vi "invert joystick cluster values.vi"(6 "Invert Z":bool, 8 "Invert Y":bool, 9 "Invert X":bool, 10 "Slide":cluster{u32, u32, u32}(slide) scale=0.0..7.0, 11 "Joystick Readings":T1) -> (3 "Joystick Readings 2":T1)   [LabVIEW 2012]
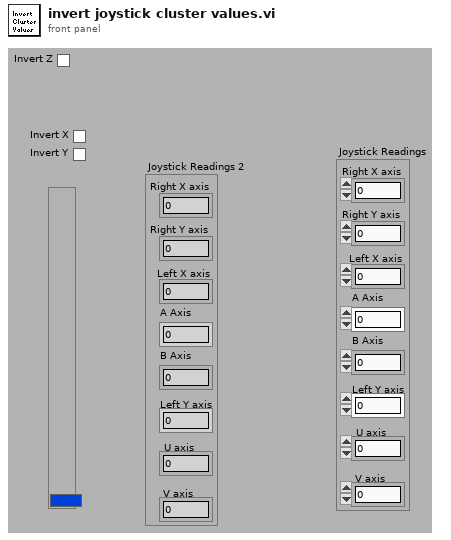
[diagram p1: front panel]
types:
  T1 = cluster{"Right X axis":i32, "Right Y axis":i32, "Left X axis":i32, "A Axis":i32, "B Axis":i32, "Left Y axis":i32, "U axis":i32, "V axis":i32}
  T2 = cluster{"Joystick Readings[0]":i32, "Joystick Readings[1]":i32, "Joystick Readings[2]":i32, "Joystick Readings[3]":i32, "Joystick Readings[4]":i32, "Joystick Readings[5]":i32, "Joystick Readings[6]":i32, "Joystick Readings[7]":i32, "Joystick Readings[8]":i32}
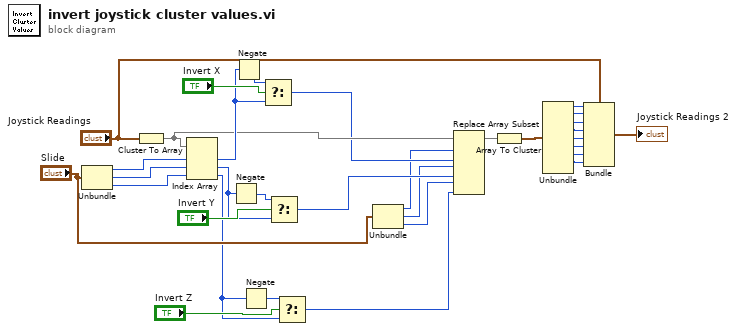
[diagram p0: block diagram]
diagram:
  n1 = Unbundle("Slide") -> (w32:u32, w31:u32, w6:u32)
  n2 = Cluster To Array(cluster="Joystick Readings") -> (array=w24:i32[])
  n3 = Index Array(array=w24, index #1=w32, index #2=w31, index #3=w6) -> (element #1=w25:i32, element #2=w27:i32, element #3=w1:i32)
  n4 = Negate(x=w27) -> (-x=w28:i32)
  n5 = Negate(x=w25) -> (-x=w26:i32)
  n6 = Negate(x=w1) -> (-x=w3:i32)
  n7 = Select(t=w26, s="Invert X", f=w25) -> (s? t:f=w23:i32)
  n8 = Select(t=w28, s="Invert Y", f=w27) -> (s? t:f=w22:i32)
  n9 = Select(t=w3, s="Invert Z", f=w1) -> (s? t:f=w4:i32)
  n10 = Unbundle("Slide") -> (w20:u32, w19:u32, w5:u32)
  n11 = Replace Array Subset(array=w24, new element #1=w23, index #1=w20, new element #2=w22, index #2=w19, new element #3=w4, index #3=w5) -> (w18:i32[])
  n12 = Array To Cluster(array=w18) -> (cluster=w17:T2)
  n13 = Unbundle(w17) -> ("Joystick Readings[0]"=w15:i32, "Joystick Readings[1]"=w14:i32, "Joystick Readings[2]"=w13:i32, "Joystick Readings[3]"=w12:i32, "Joystick Readings[4]"=w11:i32, "Joystick Readings[5]"=w10:i32, "Joystick Readings[6]"=w9:i32, "Joystick Readings[7]"=w8:i32)  [unwired: 1 out]
  n14 = Bundle(cluster="Joystick Readings", "Right X axis"=w15, "Right Y axis"=w14, "Left X axis"=w13, "A Axis"=w12, "B Axis"=w11, "Left Y axis"=w10, "U axis"=w9, "V axis"=w8) -> (→"Joystick Readings 2":T1)
